vi "Hello World.vi"() -> ()   [LabVIEW 2019]
panel:
  in  "stop":bool
  in  "message":string="Hello World!"
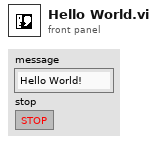
[diagram p1: front panel]
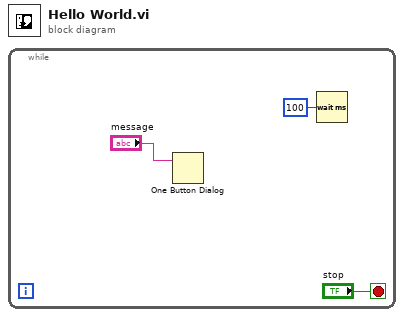
[diagram p0: block diagram]
diagram:
  n1 = while {
    stop <- "stop" stop-if-true
    n2 = One Button Dialog(message="message") -> ()  [unwired: 1 in, 1 out]
    n3 = Wait (ms)(milliseconds to wait=u32 100) -> ()  [unwired: 1 out]
  }
